vi "Doc Object[].vi"(0 "Document Class[]":refnum<class "Document.lvclass">[](array[class]), 5 "Path":path, 7 "Document Class":refnum<class "Document.lvclass">, 11 "error in (no error)":errorcluster) -> (4 "Document Class[]":refnum<class "Document.lvclass">[](array[class]), 15 "error out":errorcluster)   [LabVIEW 2016]
uses:
  source code/Document/Document.lvclass
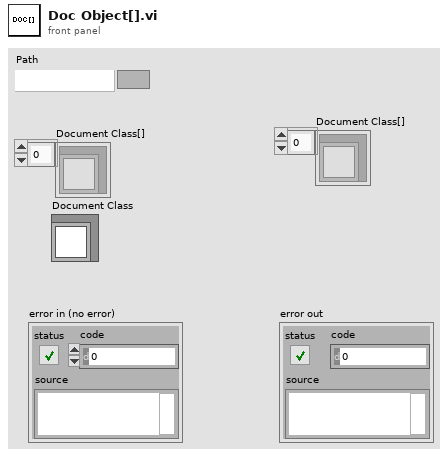
[diagram p1: front panel]
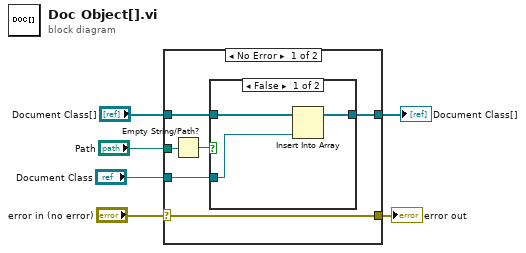
[diagram p0: block diagram]
diagram:
  n1 = case shown="No Error" "error in (no error)" {
    selector: "error in (no error)" -> [w7 w18]
    tunnel: "Path" -> [w12 _]
    tunnel: "Document Class[]" -> [w10 w17]
    tunnel: "Document Class" -> [w9 _]
    tunnel: [w8 w17] -> w3
    tunnel: [w7 w18] -> w1
    frame No Error {
      n2 = Empty String/Path?(string/path=w12) -> (empty?=w11:bool)
      n3 = case shown="False" w11 {
        tunnel: w10 -> [w15 w16]
        tunnel: w9 -> [w14 _]
        tunnel: [w13 w16] -> w8
        frame False {
          n4 = Insert Into Array(array=w15, new element=w14) -> (w13:refnum<class "Document.lvclass">[])  [unwired: 1 in]
        }
        frame True {
        }
      }
    }
    frame Error {
    }
  }
  "Document Class[]" <- w3
  "error out" <- w1
